vi "Untitled 1.vi"() -> ()   [LabVIEW 2020]
panel:
  out "s? t:f":dbl[](array[numeric])
  in  "Boolean":bool
  out "String":string
  in  "'":i32=1
  out "Slide 2":dbl(slide) scale=0.0..300.0
  in  "Array 2  1":dbl
  in  "Array 2   0":dbl
  out "Numeric 3":i32
  in  "Array 1   1":dbl
  in  "Array 1   0":dbl
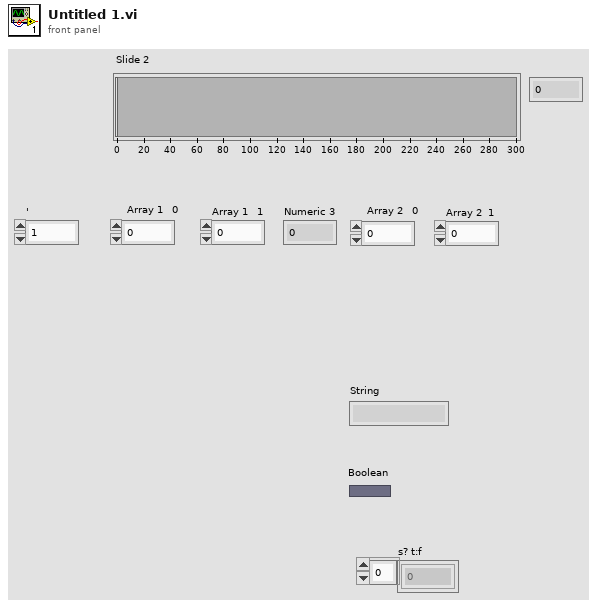
[diagram p1: front panel]
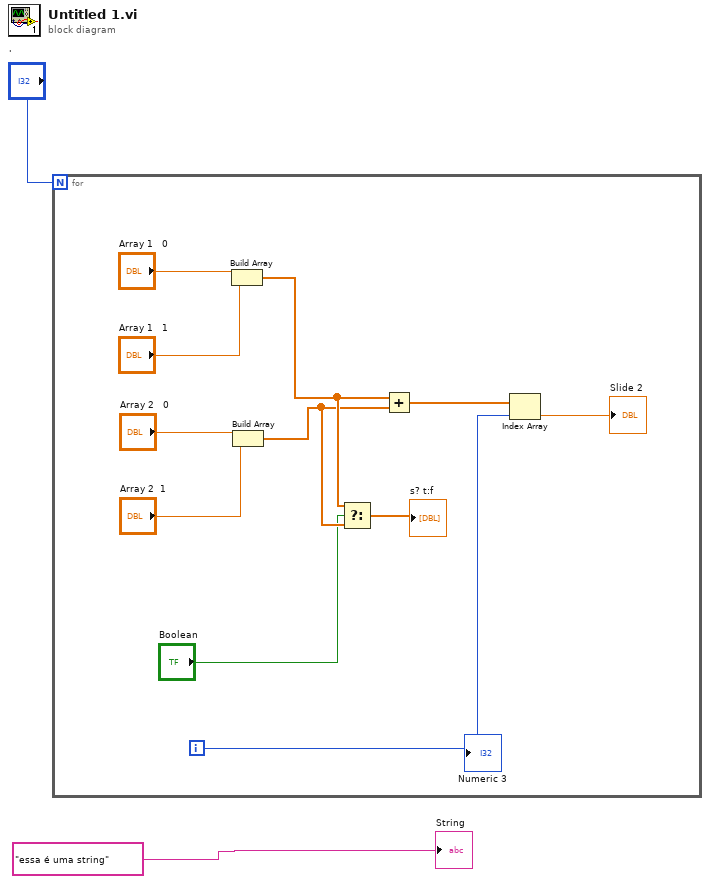
[diagram p0: block diagram]
diagram:
  n1 = for {
    N: "'" -> [_]
    i -> [w8]
    n2 = Build Array("Array 1   0", "Array 1   1") -> (w6:dbl[])
    n3 = Build Array("Array 2   0", "Array 2  1") -> (w5:dbl[])
    n4 = Select(t=w6, s="Boolean", f=w5) -> (s? t:f=→"s? t:f":dbl[])
    n5 = Add(x=w6, y=w5) -> (x+y=w9:dbl[])
    n6 = Index Array(array=w9, index=w8) -> (element=→"Slide 2":dbl)
    "Numeric 3" <- w8
  }
  "String" <- "essa é uma string"
